vi "Handle Incoming Packets.vi"(8 "error in (no error)":errorcluster, 10 "Incoming Packets":u8[](array[numeric]) format="%08b", 11 "ControlPacket in":refnum<class "ControlPacket.lvclass">) -> (0 "error out":errorcluster, 1 "Complete?":bool=TRUE, 2 "Remaining Packets":u8[](array[numeric]) format="%08b", 3 "ControlPacket out":refnum<class "ControlPacket.lvclass">)   [LabVIEW 2013, in "ControlPacket.lvclass"]
uses:
  ControlPacket.lvclass
  ControlPacket.lvclass/ControlPacket.ctl
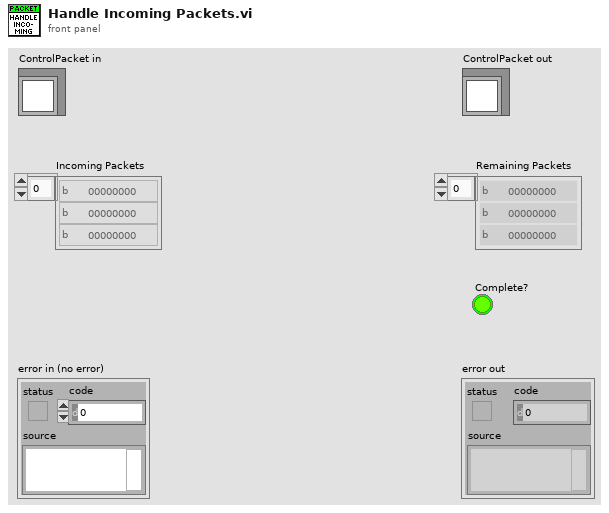
[diagram p1: front panel]
types:
  T1 = enum16{"Extract Length", "Extract Variable Header", "Append Payload", "Exit"}
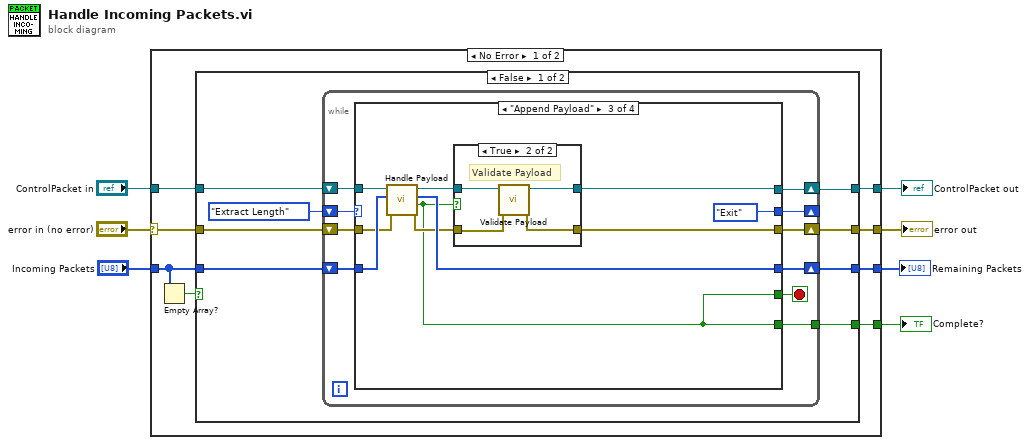
[diagram p0: block diagram]
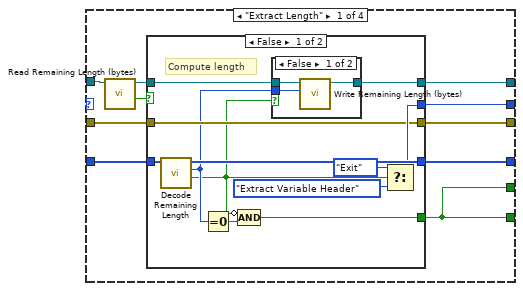
[diagram p2: hidden frame]
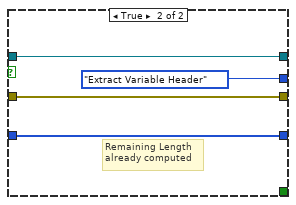
[diagram p4: hidden frame]
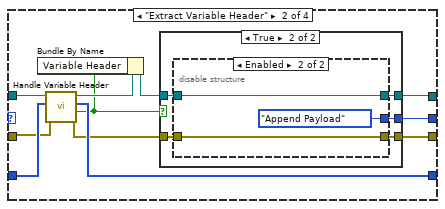
[diagram p5: hidden frame]
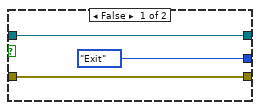
[diagram p6: hidden frame]
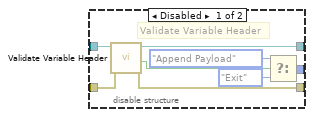
[diagram p7: hidden frame]
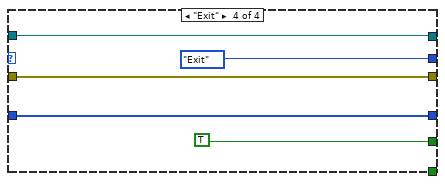
[diagram p9: hidden frame]
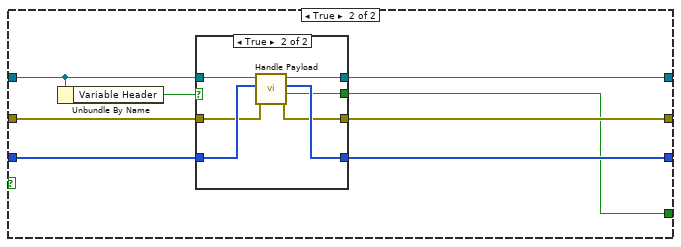
[diagram p10: hidden frame]
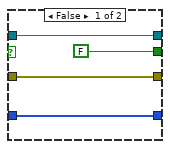
[diagram p11: hidden frame]
diagram:
  n1 = case shown="No Error" "error in (no error)" {
    selector: "error in (no error)" -> [w12 w136]
    tunnel: [w11 w136] -> w6
    tunnel: [w10 w135] -> w4
    tunnel: "ControlPacket in" -> [w15 w135]
    tunnel: "Incoming Packets" -> [w14 w134]
    tunnel: [w9 w134] -> w2
    tunnel: [w8 _] -> w1
    frame No Error {
      n2 = Empty Array?(array=w14) -> (empty?=w13:bool)
      n3 = case shown="False" w13 {
        tunnel: w15 -> [w17 w115]
        tunnel: w14 -> [w23 w119]
        tunnel: w12 -> [w18 w120]
        tunnel: [w21 w117] -> w11
        tunnel: [w22 w121] -> w10
        tunnel: [w20 w118] -> w9
        tunnel: [w19 w116] -> w8
        frame False {
          n4 = while {
            shift-right: [w30] -> w22
            shift-left: w17 -> [w33]
            shift-right: [w29] -> w21
            shift-left: w18 -> [w31]
            shift-right: [w28] -> w20
            shift-left: w23 -> [w32]
            shift-right: [w26] -> _
            shift-left: T1."Extract Length" -> [w27]
            tunnel: [w24] -> w19
            stop <- w25 stop-if-true
            n5 = case shown="\"Append Payload\"" w27 {
              tunnel: w33 -> [w43 w74 w103 w114]
              tunnel: w32 -> [w41 w73 w102 w110]
              tunnel: w31 -> [w40 w71 w100 w111]
              tunnel: [w39 w68 w97 w114] -> w30
              tunnel: [w38 w66 w94 w111] -> w29
              tunnel: [w37 w72 w101 w110] -> w28
              tunnel: [w36 w64 T1."Exit" T1."Exit"] -> w26
              tunnel: [w35 _ w95 TRUE] -> w25
              tunnel: [w35 _ w95 _] -> w24
              frame "Extract Length" {
                n6 = call "Read Remaining Length (bytes).vi"("ControlPacket in"=w43) -> ("Length"=w34:bool, "ControlPacket out"=w42:refnum<class "ControlPacket.lvclass">)  [unwired: 8 in, 1 out]
                n7 = case shown="False" w34 {
                  tunnel: w42 -> [w53 w63]
                  tunnel: [w52 w63] -> w39
                  tunnel: w41 -> [w55 w62]
                  tunnel: [w54 w62] -> w37
                  tunnel: w40 -> [w50 w61]
                  tunnel: [w50 w61] -> w38
                  tunnel: [w51 T1."Extract Variable Header"] -> w36
                  tunnel: [w47 _] -> w35
                  frame False {
                    # "Compute length"
                    n8 = call "Decode Remaining Length.vi"("Packet w/o 1st byte"=w55) -> ("Malformed Remaining Length"=w44:bool, "Remaining Length (bytes)"=w49:u32, "Remaining Packet"=w54:u8[])  [unwired: 8 in]
                    n9 = Equal To 0?(x=w49) -> (x = 0?=w48:bool)
                    n10 = Compound Arithmetic op=AND(invert w44, w48) -> (w47:bool)
                    n11 = case shown="False" w44 {
                      tunnel: w53 -> [w58 w59]
                      tunnel: [w57 w59] -> w52
                      tunnel: w49 -> [w56 _]
                      frame False {
                        n12 = call "Write Remaining Length (bytes).vi"("Remaining Length (bytes)"=w56, "ControlPacket in"=w58) -> ("ControlPacket out"=w57:refnum<class "ControlPacket.lvclass">)  [unwired: 9 in]
                      }
                      frame True {
                      }
                    }
                    n13 = Select(t=T1."Exit", s=w44, f=T1."Extract Variable Header") -> (s? t:f=w51:T1)
                  }
                  frame True {
                    # "Remaining Length\nalready computed"
                  }
                }
              }
              frame "Extract Variable Header" {
                n14 = call-dynamic "Handle Variable Header.vi"("error in (no error)"=w71, "Incoming Packets"=w73, "ControlPacket in"=w74) -> ("error out"=w67:errorcluster, "Variable Header Complete?"=w65:bool, "Remaining Packets"=w72:u8[], "ControlPacket out"=w70:refnum<class "ControlPacket.lvclass">)  [unwired: 5 in]
                n15 = Bundle By Name(cluster=w70, "Variable Header"=w65) -> (w69:refnum<class "ControlPacket.lvclass">)
                n16 = case shown="True" w65 {
                  tunnel: w69 -> [w77 w82]
                  tunnel: [w77 w81] -> w68
                  tunnel: w67 -> [w76 w80]
                  tunnel: [w76 w79] -> w66
                  tunnel: [T1."Exit" w78] -> w64
                  frame False {
                  }
                  frame True {
                    n17 = disable-structure shown="Enabled" {
                      disable-tunnel: w82 -> [w90 w93]
                      disable-tunnel: [w89 w93] -> w81
                      disable-tunnel: w80 -> [w88 w92]
                      disable-tunnel: [w87 w92] -> w79
                      disable-tunnel: [w85 T1."Append Payload"] -> w78
                      frame Disabled {
                        # "Validate Variable Header"
                        n18 = call-dynamic "Validate Variable Header.vi"("error in (no error)"=w88, "ControlPacket in"=w90) -> ("error out"=w87:errorcluster, "valid?"=w84:bool, "ControlPacket out"=w89:refnum<class "ControlPacket.lvclass">)  [unwired: 7 in]
                        n19 = Select(t=T1."Append Payload", s=w84, f=T1."Exit") -> (s? t:f=w85:T1)
                      }
                      frame Enabled {
                      }
                    }
                  }
                }
              }
              frame "Append Payload" {
                n20 = call "Handle Payload.vi"("error in (no error)"=w100, "Incoming Packets"=w102, "ControlPacket in"=w103) -> ("error out"=w96:errorcluster, "Payload Complete?"=w95:bool, "Remaining Packets"=w101:u8[], "ControlPacket out"=w98:refnum<class "ControlPacket.lvclass">)  [unwired: 5 in]
                n21 = case shown="True" w95 {
                  tunnel: w98 -> [w105 w109]
                  tunnel: [w105 w108] -> w97
                  tunnel: w96 -> [w104 w107]
                  tunnel: [w104 w106] -> w94
                  frame False {
                  }
                  frame True {
                    # "Validate Payload"
                    n22 = call-dynamic "Validate Payload.vi"("error in (no error)"=w107, "ControlPacket in"=w109) -> ("error out"=w106:errorcluster, "ControlPacket out"=w108:refnum<class "ControlPacket.lvclass">)  [unwired: 7 in, 1 out]
                  }
                }
              }
              frame "Exit" {
              }
            }
          }
        }
        frame True {
          n23 = Unbundle By Name(w115) -> ("Variable Header"=w122:bool)
          n24 = case shown="True" w122 {
            tunnel: w115 -> [w126 w133]
            tunnel: [w126 w132] -> w121
            tunnel: w120 -> [w124 w129]
            tunnel: w119 -> [w125 w131]
            tunnel: [w125 w130] -> w118
            tunnel: [w124 w128] -> w117
            tunnel: [FALSE w127] -> w116
            frame False {
            }
            frame True {
              n25 = call "Handle Payload.vi"("error in (no error)"=w129, "Incoming Packets"=w131, "ControlPacket in"=w133) -> ("error out"=w128:errorcluster, "Payload Complete?"=w127:bool, "Remaining Packets"=w130:u8[], "ControlPacket out"=w132:refnum<class "ControlPacket.lvclass">)  [unwired: 5 in]
            }
          }
        }
      }
    }
    frame Error {
    }
  }
  "error out" <- w6
  "ControlPacket out" <- w4
  "Remaining Packets" <- w2
  "Complete?" <- w1
